vi "Decode Robots Referee.vi"(8 "error in":errorcluster, 9 "array":u8[](array[numeric]), 10 "Key":i32=5) -> (0 "error out":errorcluster, 1 "array w/ subset deleted out":u8[](array[numeric]), 3 "team info":T1)   [LabVIEW 2016]
uses:
  SSL Referee Team Info.ctl
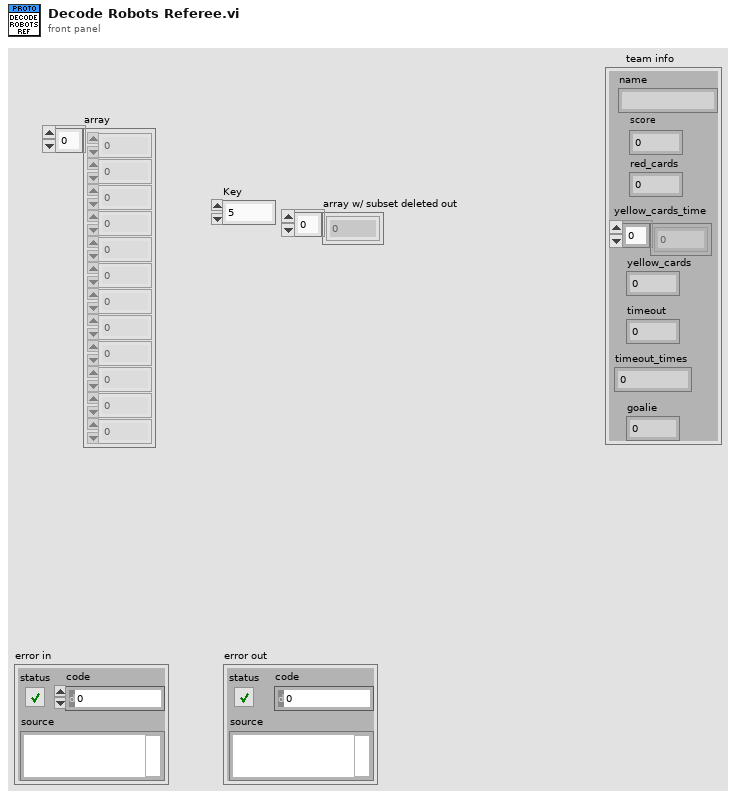
[diagram p1: front panel]
types:
  T1 = typedef "SSL Referee Team Info.ctl" = cluster{"name":string, "score":u32, "red_cards":u32, "yellow_cards_time":u32[], "yellow_cards":u32, "timeout":u32, "timeout_times":u32, "goalie":u32}
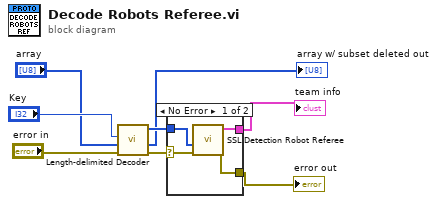
[diagram p0: block diagram]
diagram:
  n1 = call "Length-delimited Decoder.vi"("error in (no error)"="error in", "Array"="array", "Key"="Key") -> ("error out"=w8:errorcluster, "array w/ subset deleted"=→"array w/ subset deleted out":u8[], "Length-delimited"=w7:u8[])  [unwired: 5 in, 1 out]
  n2 = case shown="No Error" w8 {
    selector: w8 -> [w11 w13]
    tunnel: [w12 w13] -> w6
    tunnel: w7 -> [w10 _]
    tunnel: [w9 _] -> w5
    frame No Error {
      n3 = call "SSL Detection Robot Referee.vi"("error in"=w11, "Array"=w10) -> ("error out"=w12:errorcluster, "output cluster"=w9:T1)  [unwired: 7 in, 1 out]
    }
    frame Error {
    }
  }
  "error out" <- w6
  "team info" <- w5
